vi "4_1_2.vi"() -> ()   [LabVIEW 2025, in "2022.lvlib"]
uses:
  2022.lvlib
  e0d1e511-853d-49ec-a1d4-7fdb9e36fbb4.vi
panel:
  out "size(s) 2":i32
  out "Array 4":bool[](array[boolean])
  out "size(s)":i32
  out "Array 3":bool[](array[boolean])
  out "x .or. y?":bool
  out "intersection":set{i32}(c389)
  out "Array 2":i32[](array[numeric])
  out "Array":i32[](array[numeric])
  out "output 4":i32
  out "output 3":i32
  out "output 2":i32
  out "output 1":i32
  out "subarray":string[](array[string])
  out "array":string[][](array[string])
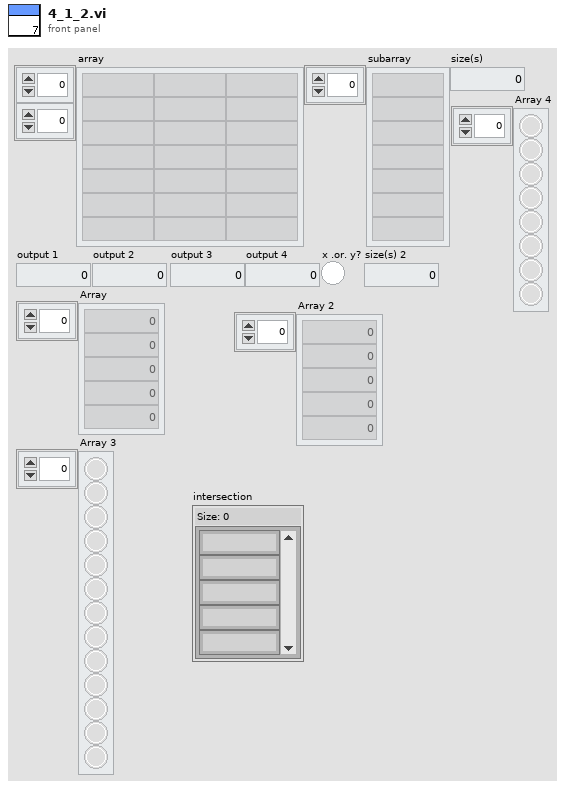
[diagram p1: front panel]
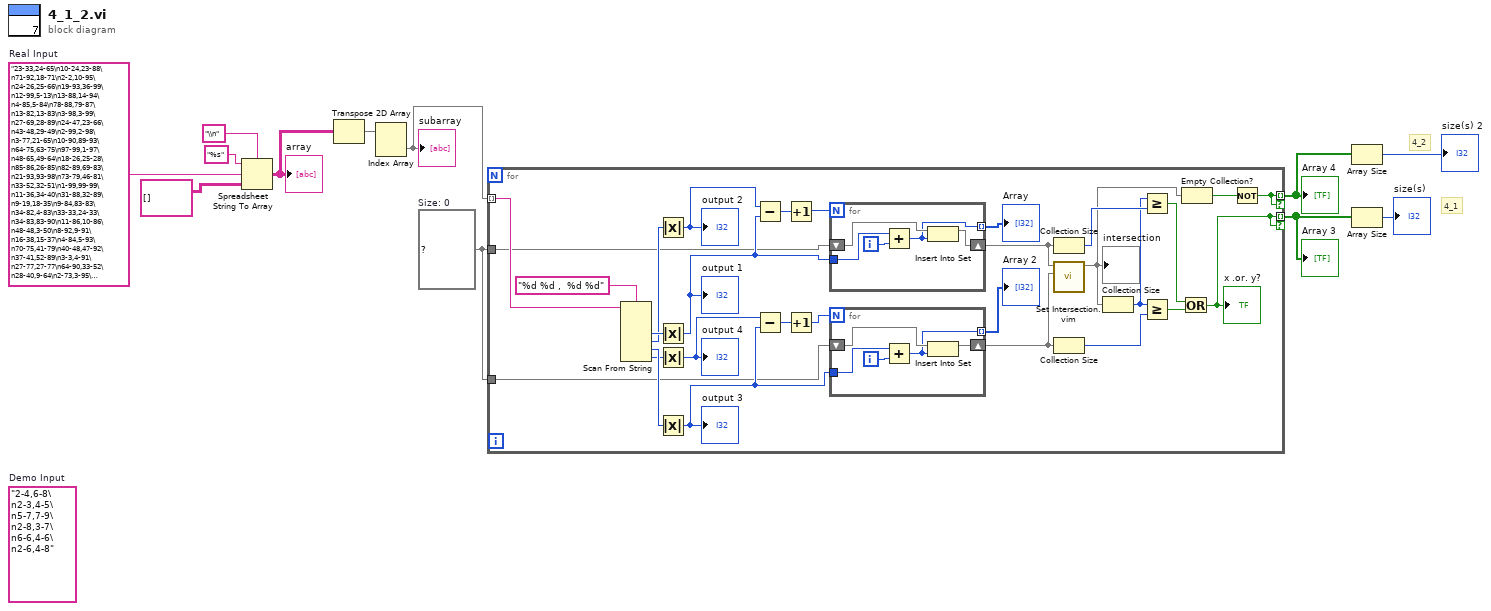
[diagram p0: block diagram]
diagram:
  w6 = set{i32} {}  # Size: 0
  w1 = "23-33,24-65\n10-24,23-88\n71-92,18-71\n2-2,10-95\n24-26,25-66\n19-93,36-99\n12-99,5-13\n13-88,14-94\n4-85,5-84\n78-88,79-87\n13-82,13-83\n3-98,3-99\n27-69,28-89\n24-47,23-66\n43-48,29-49\n2-99,2-98\n3-77,21-65\n10-90,89-93\n64-75,63-75\n97-99,1-97\n48-65,49-64\n18-26,25-28\n85-86,26-85\n82-89,69-83\n21-93,93-98\n73-79,46-81\n33-52,32-51\n1-99,99-99\n11-36,34-40\n31-88,32-89\n9-19,18-35\n9-84,83-83\n34-82,4-83\n33-33,24-33\n34-83,83-90\n11-86,10-86\n48-48,3-50\n8-92,9-91\n16-38,15-37\n4-84,5-93\n70-75,41-79\n40-48,47-92\n37-41,52-89\n3-3,4-91\n27-77,27-77\n64-90,33-52\n28-40,9-64\n2-73,3-95\n17-94,7-75\n6-71,7-71\n11-69,10-70\n4-40,4-40\n9-54,30-44\n92-93,4-92\n62-63,63-67\n7-34,16-34\n54-55,31-54\n12-90,11-91\n11-13,12-53\n10-73,9-64\n13-18,13-84\n6-82,16-81\n52-78,18-53\n22-82,23-74\n90-91,3-90\n92-93,70-93\n18-44,19-45\n20-20,20-67\n31-93,76-93\n25-86,86-86\n6-73,5-94\n75-84,74-86\n50-51,50-51\n56-86,57-86\n18-81,13-18\n3-9,8-93\n31-36,34-34\n19-88,18-87\n10-95,54-79\n83-85,66-86\n32-68,31-49\n14-97,12-99\n42-42,42-53\n27-32,28-69\n96-98,15-96\n25-49,25-48\n71-81,15-92\n19-83,15-19\n14-99,6-14\n52-90,53-94\n5-98,85-96\n18-30,10-15\n4-86,4-98\n54-55,30-78\n85-99,62-86\n10-99,10-98\n4-96,5-95\n6-59,7-18\n6-86,1-7\n28-85,5-84\n3-82,2-82\n73-92,87-87\n2-3,2-89\n4-5,4-8\n21-96,69-97\n89-90,4-89\n28-79,29-80\n35-58,40-48\n96-96,3-97\n17-27,16-96\n7-99,8-94\n26-92,25-92\n17-24,17-25\n44-44,40-47\n57-64,57-65\n60-91,59-79\n23-79,22-71\n34-37,31-70\n22-60,22-59\n44-99,98-98\n9-57,49-55\n61-64,33-62\n15-68,4-15\n53-55,34-55\n13-13,9-15\n2-43,3-81\n17-56,16-99\n1-4,3-92\n76-77,73-83\n2-97,2-96\n44-45,44-55\n8-89,8-97\n23-73,22-88\n23-90,79-93\n23-87,86-91\n3-45,17-44\n7-99,8-98\n92-97,14-92\n85-89,59-90\n7-8,7-89\n5-90,49-89\n28-30,29-63\n38-61,38-60\n32-98,5-75\n22-87,71-76\n5-85,5-88\n16-96,18-88\n39-51,40-90\n21-21,19-23\n22-55,15-56\n1-75,35-59\n13-84,12-85\n11-83,23-27\n11-98,11-97\n35-92,34-92\n8-96,8-30\n48-72,33-60\n9-83,10-82\n97-97,10-98\n5-7,9-98\n1-44,3-43\n7-85,8-85\n12-32,12-52\n1-86,86-86\n3-63,4-63\n3-83,83-91\n74-88,38-74\n92-95,6-98\n11-19,10-20\n6-94,7-94\n39-90,38-42\n60-92,61-92\n43-94,44-98\n23-98,22-99\n31-41,27-32\n9-79,9-78\n63-64,11-64\n82-82,83-98\n78-79,77-78\n19-63,4-27\n26-62,27-44\n91-91,91-93\n16-94,31-93\n23-25,24-99\n78-79,11-78\n30-30,29-31\n34-85,35-84\n4-78,4-5\n42-84,43-85\n39-87,40-86\n49-84,50-84\n67-67,7-67\n38-38,62-67\n2-83,3-82\n14-33,32-68\n18-76,17-75\n68-77,68-76\n4-97,53-73\n53-97,54-96\n53-55,54-98\n35-95,75-83\n2-3,2-78\n3-97,15-96\n26-87,26-92\n4-10,9-48\n3-89,22-96\n10-85,10-84\n1-93,2-2\n24-37,37-62\n32-68,48-53\n33-96,95-97\n9-26,14-31\n16-66,13-14\n85-86,78-85\n65-82,64-81\n5-85,31-49\n47-88,59-91\n34-71,70-76\n14-14,14-14\n45-46,45-97\n63-73,63-64\n16-54,17-53\n87-88,51-87\n20-79,19-98\n3-96,2-95\n86-86,60-86\n82-82,67-82\n12-35,11-35\n15-31,26-52\n1-2,1-99\n3-96,2-2\n91-97,11-92\n41-89,42-96\n62-64,41-65\n54-54,16-55\n28-41,40-97\n15-89,89-90\n50-71,55-70\n30-66,30-93\n89-92,84-89\n25-27,26-84\n59-91,60-91\n4-11,4-98\n5-48,10-44\n53-80,77-79\n20-21,10-20\n14-86,14-85\n32-70,33-69\n94-94,26-95\n5-57,5-97\n38-50,38-92\n48-50,49-51\n13-98,12-98\n90-95,24-88\n90-94,67-91\n1-11,10-91\n48-59,59-91\n26-68,31-55\n15-56,21-57\n6-69,7-69\n6-8,5-95\n32-93,33-94\n13-73,14-42\n1-4,3-98\n30-62,29-62\n57-64,61-99\n12-27,11-46\n28-99,98-98\n7-83,8-92\n56-77,56-76\n30-89,31-51\n69-83,37-72\n11-78,11-65\n61-61,60-62\n38-65,65-66\n20-44,21-97\n39-76,40-75\n10-94,11-93\n33-90,89-96\n23-77,22-78\n63-86,62-73\n42-81,35-43\n34-91,34-55\n12-97,4-13\n1-98,1-97\n23-72,24-73\n14-99,13-99\n17-97,18-96\n65-85,14-66\n68-77,67-69\n8-96,9-9\n28-57,29-56\n14-26,14-26\n6-72,6-72\n49-49,1-48\n4-65,65-65\n53-92,54-91\n48-87,15-48\n51-54,20-72\n65-75,64-64\n4-92,3-93\n42-70,30-98\n15-71,14-15\n29-62,28-63\n6-92,6-93\n37-84,83-83\n1-99,23-98\n23-82,24-88\n2-60,61-74\n3-5,17-93\n50-63,51-62\n51-55,52-52\n30-82,5-83\n5-77,4-42\n44-99,3-99\n18-81,5-18\n2-32,32-32\n50-59,58-87\n23-30,24-40\n70-70,9-71\n40-62,49-62\n2-29,1-3\n48-69,48-49\n48-48,47-93\n5-42,17-41\n11-95,12-92\n9-66,8-65\n32-84,33-84\n16-69,15-99\n12-96,9-12\n69-91,68-70\n14-69,15-81\n96-99,50-96\n35-62,35-61\n6-22,22-60\n20-76,73-74\n4-21,4-22\n22-30,21-76\n5-90,1-6\n82-96,82-95\n18-31,19-71\n29-56,50-59\n11-21,1-61\n15-76,30-81\n1-1,2-83\n11-90,90-91\n40-90,40-41\n68-83,68-83\n25-81,25-81\n87-88,22-87\n31-65,32-64\n17-90,16-90\n11-65,11-12\n35-60,36-93\n5-93,4-94\n28-29,27-75\n12-38,37-45\n39-46,32-44\n12-89,12-97\n4-54,52-52\n5-94,94-94\n30-31,29-31\n18-82,74-76\n80-80,59-81\n3-65,54-54\n20-31,19-23\n82-87,32-82\n41-41,41-42\n6-6,6-81\n2-98,98-98\n84-94,6-95\n29-89,28-92\n27-30,28-34\n5-86,4-86\n32-96,50-96\n28-93,69-90\n75-75,27-82\n9-30,30-36\n76-76,61-77\n74-80,11-74\n48-61,48-60\n64-98,64-99\n83-87,5-88\n23-25,25-98\n55-55,39-55\n5-36,5-36\n45-57,46-85\n4-86,3-85\n19-58,20-58\n25-83,14-26\n27-74,27-27\n17-18,17-45\n81-88,62-84\n84-96,21-85\n3-81,1-2\n54-93,1-94\n1-1,3-66\n69-78,49-78\n47-93,47-93\n13-13,13-66\n18-78,18-73\n11-20,15-18\n52-99,51-99\n2-57,1-58\n9-97,10-97\n80-80,24-80\n33-77,34-47\n68-75,67-73\n20-95,19-95\n4-99,5-98\n8-85,7-85\n42-80,66-82\n22-47,31-47\n22-26,24-24\n4-98,38-44\n92-94,92-95\n82-92,71-94\n6-10,1-5\n3-92,1-92\n72-76,71-74\n6-69,7-69\n25-75,26-66\n15-51,15-63\n14-99,14-98\n7-89,6-70\n58-66,62-85\n7-11,15-23\n42-62,42-63\n1-4,4-91\n1-3,3-97\n49-79,48-80\n15-95,16-77\n6-99,5-99\n6-79,8-27\n47-69,46-68\n20-21,24-96\n13-71,60-92\n69-94,36-69\n66-86,33-67\n34-47,34-47\n4-4,4-93\n22-68,68-68\n42-90,43-90\n74-74,74-94\n3-72,3-62\n63-75,64-67\n16-48,7-48\n2-89,3-99\n2-98,3-97\n41-94,42-95\n45-93,44-98\n16-18,17-64\n69-70,47-69\n2-93,93-94\n65-94,66-95\n54-56,55-57\n5-92,2-92\n48-92,28-45\n67-68,48-67\n7-12,6-8\n7-8,6-8\n94-99,16-95\n13-49,14-48\n25-48,48-48\n6-51,7-18\n46-83,15-97\n34-57,34-58\n16-89,9-17\n41-74,41-42\n13-32,13-97\n90-99,99-99\n7-99,7-98\n78-79,63-78\n4-98,64-79\n49-75,50-80\n40-75,40-52\n14-72,6-14\n5-91,91-91\n27-55,27-27\n20-22,27-37\n35-71,34-96\n2-52,1-1\n3-87,2-87\n2-70,36-69\n38-90,39-89\n67-79,67-80\n5-77,77-78\n26-32,2-34\n10-43,43-85\n55-84,84-85\n24-59,24-58\n43-49,44-48\n60-81,59-80\n52-91,91-92\n44-62,42-63\n3-96,3-97\n29-45,30-45\n64-92,6-93\n89-96,4-90\n71-91,71-90\n50-64,60-63\n49-88,49-89\n18-98,18-90\n30-74,72-77\n32-88,4-76\n22-58,22-23\n5-71,5-18\n8-90,7-98\n4-78,4-79\n54-87,54-55\n3-91,3-92\n14-92,89-91\n41-95,42-42\n74-75,53-77\n12-90,3-12\n5-50,3-51\n27-67,66-68\n10-42,24-38\n20-79,20-81\n10-78,78-97\n26-47,35-46\n34-82,34-63\n2-94,3-98\n19-87,19-87\n4-42,6-90\n13-49,12-14\n75-75,3-76\n55-70,54-56\n86-92,85-93\n31-38,28-46\n7-90,6-91\n33-72,32-50\n22-46,45-99\n45-53,46-51\n90-91,6-90\n13-87,14-45\n41-95,14-42\n90-95,76-95\n51-70,15-89\n15-49,25-95\n15-15,15-98\n20-88,14-33\n2-67,67-70\n88-93,78-96\n77-91,53-84\n53-88,52-98\n24-96,25-25\n40-40,26-40\n3-15,9-25\n35-99,36-97\n61-61,4-62\n5-95,6-6\n52-56,52-95\n22-30,23-23\n40-44,43-63\n13-16,5-14\n18-90,89-89\n5-88,4-88\n78-83,82-82\n6-80,1-1\n15-31,14-32\n13-96,13-13\n68-76,68-69\n56-67,67-90\n24-92,92-93\n16-29,17-90\n2-99,1-90\n12-75,1-13\n21-91,20-90\n1-99,11-97\n94-94,25-95\n2-91,3-92\n95-95,2-95\n2-99,1-97\n28-98,27-29\n6-26,2-67\n20-58,19-71\n32-87,49-86\n13-57,14-56\n2-55,11-44\n13-61,12-61\n33-81,80-80\n39-91,41-44\n40-93,39-47\n83-95,40-93\n20-79,24-78\n52-93,6-94\n96-96,3-97\n44-55,36-87\n43-44,13-43\n19-99,19-98\n6-17,17-97\n91-99,88-91\n31-51,52-77\n1-97,1-2\n26-86,26-87\n50-53,40-81\n40-89,89-93\n78-83,1-79\n9-89,8-73\n6-38,7-21\n19-20,18-21\n97-97,35-97\n28-57,20-28\n3-86,86-87\n53-53,2-52\n59-99,60-99\n75-84,76-95\n20-93,21-94\n29-29,29-30\n34-92,15-58\n11-58,11-59\n11-11,10-98\n19-77,77-77\n38-56,38-71\n83-86,12-88\n8-73,5-6\n5-7,7-93\n18-79,19-72\n4-99,2-2\n5-82,5-81\n24-37,37-95\n11-63,9-12\n6-99,7-98\n92-92,91-91\n58-91,2-95\n23-98,24-59\n2-90,3-89\n54-71,1-81\n22-98,48-97\n14-49,13-76\n5-52,6-89\n6-88,76-86\n3-85,6-97\n87-94,86-88\n30-46,31-45\n63-95,9-97\n19-94,94-98\n71-75,72-74\n48-89,49-89\n27-52,52-54\n21-99,41-94\n5-96,3-5\n40-69,38-40\n74-99,73-98\n6-31,22-85\n13-76,12-75\n29-74,29-74\n10-86,11-86\n40-41,33-40\n63-94,29-94\n55-85,55-55\n14-20,18-19\n52-78,1-79\n92-96,7-92\n12-89,14-57\n32-49,49-82\n36-63,43-62\n20-94,41-93\n79-95,7-97\n5-60,5-22\n29-93,28-93\n18-68,18-67\n12-37,13-36\n12-64,12-46\n1-99,2-2\n61-92,61-82\n14-16,15-68\n68-83,67-77\n24-93,93-93\n33-99,32-33\n93-93,11-94\n27-37,26-37\n7-31,6-31\n1-45,2-67\n5-99,5-99\n20-21,18-22\n22-89,23-88\n53-58,53-56\n48-91,48-86\n11-11,10-12\n33-50,50-81\n11-47,7-20\n51-71,71-72\n15-89,15-88\n6-90,2-15\n7-88,18-91\n4-98,4-98\n9-19,3-19\n29-58,57-83\n16-34,15-33\n13-50,12-89\n17-60,17-17\n90-94,91-98\n52-77,52-76\n97-99,5-97\n42-86,53-76\n4-7,19-56\n23-63,2-41\n15-43,43-44\n19-23,22-97\n47-48,45-49\n31-73,32-73\n57-72,21-38\n54-97,53-96\n2-29,3-64\n53-79,13-77\n63-77,4-63\n94-94,4-95\n5-44,4-98\n5-99,4-98\n31-96,32-96\n44-89,43-90\n1-63,2-63\n31-60,8-32\n48-88,55-62\n36-85,35-85\n7-98,97-97\n3-52,4-99\n19-57,1-20\n65-96,66-97\n61-95,43-62\n4-94,93-93\n14-97,58-96\n26-46,6-47\n79-96,81-95\n30-88,30-87\n27-97,26-96\n24-88,24-25\n27-95,28-51\n22-24,23-76\n40-44,44-52\n4-37,3-38\n6-7,4-8\n22-24,16-25\n59-73,58-73\n2-14,3-40\n20-65,65-65\n58-87,58-86\n99-99,26-98\n10-17,16-91\n52-71,59-70\n3-87,2-87\n22-95,95-96\n55-55,10-54\n52-84,82-96\n5-82,81-81\n9-95,7-7\n53-88,88-90\n5-6,5-63\n11-68,10-85\n8-12,10-11\n40-92,43-49\n19-35,20-34\n44-46,45-85\n10-25,12-26\n63-85,54-80\n10-97,91-94\n41-50,40-42\n7-72,8-71\n1-15,12-92\n22-93,54-99\n82-94,30-83\n7-89,6-89\n6-69,5-7\n8-25,24-24\n8-47,8-47\n21-25,24-92\n81-81,81-86\n6-15,44-68\n82-82,34-82\n29-86,2-87\n37-54,20-57\n56-97,1-96\n65-65,6-65\n4-81,5-82\n78-85,37-78\n18-99,19-97\n31-97,34-96\n41-58,40-77\n11-96,10-97\n18-35,7-24\n5-75,3-74\n2-53,15-47\n9-17,9-85\n20-26,21-26\n23-70,67-68\n23-72,23-73\n36-81,9-93\n25-76,25-26\n77-77,46-77\n78-98,78-87\n91-91,14-92\n22-92,21-93\n3-3,3-87\n99-99,61-99\n18-28,19-29\n44-45,19-44\n17-60,11-17\n35-97,36-36\n58-58,11-58\n24-62,23-63\n18-56,55-81\n7-31,8-30\n60-61,1-65\n8-99,7-31\n2-4,5-6\n4-93,48-92\n2-87,1-98\n3-75,3-4\n1-53,53-54\n57-73,57-68\n11-60,2-61\n51-70,43-52\n4-33,3-34\n29-68,67-68\n75-86,28-71\n4-84,3-83\n12-96,51-96\n30-98,71-94\n54-62,60-62\n13-66,14-86\n14-42,12-43\n47-69,48-69\n58-89,86-96\n27-96,27-95\n6-66,6-16\n2-30,1-37\n27-91,27-38\n46-52,45-49\n9-64,8-75\n53-92,54-93\n35-91,35-72\n66-91,91-97\n46-81,49-81\n3-90,1-3\n53-54,52-56\n4-92,3-5\n42-84,42-77\n1-3,2-95\n8-73,9-90\n17-69,16-70\n9-20,2-10\n97-99,96-97\n1-86,2-91\n17-66,9-95\n9-10,9-97\n19-40,39-54\n5-94,5-91\n33-33,18-34\n2-3,2-3\n22-66,21-84\n37-90,37-81\n6-93,6-93\n64-81,65-78\n57-59,57-67\n69-94,68-68\n39-97,38-98\n74-79,71-79\n2-80,41-80\n5-91,28-89\n1-97,2-97\n24-61,25-94\n76-81,76-97\n48-56,48-49\n25-81,7-12\n42-99,41-41\n45-60,46-59\n19-85,57-84\n8-8,7-98\n14-53,13-54\n17-82,69-84\n73-86,24-90\n78-80,6-78\n2-76,3-26\n1-33,33-89\n12-48,48-75\n25-87,21-88\n22-68,22-71\n2-91,1-91\n59-79,7-60\n6-70,4-4\n47-94,27-94\n23-50,10-49\n2-85,2-83\n2-96,7-96\n21-93,22-92\n27-67,28-67\n32-38,32-33\n15-94,93-94\n36-74,36-37\n33-84,43-83\n5-98,2-2\n1-93,2-92\n37-97,42-70\n81-82,21-81\n14-94,13-15\n5-45,4-87\n44-96,45-95\n2-7,6-14\n14-73,25-77\n83-83,84-99\n13-62,21-73\n91-98,22-91\n19-96,86-93\n5-78,6-77\n3-97,4-98\n8-54,17-83\n9-94,10-10\n36-96,35-37\n8-93,7-98\n48-60,48-61\n17-97,9-18\n73-87,74-88\n19-63,19-63\n21-73,20-74\n1-89,26-89\n44-50,48-55\n43-70,70-71\n5-14,6-63\n23-82,22-94\n20-67,18-94\n36-52,47-51\n10-84,9-83\n18-96,18-71\n3-64,4-65\n4-7,6-89\n62-89,73-99\n4-92,3-5\n3-62,45-59\n9-98,10-97\n12-80,12-89\n14-15,18-85\n7-18,6-23\n14-70,15-24\n24-52,21-78\n63-92,32-93\n47-91,42-48\n16-91,91-95\n31-66,30-65\n52-91,5-91\n85-85,11-86\n22-69,68-68\n11-58,10-21\n47-76,42-47\n63-64,43-66\n17-29,4-66\n19-19,18-86\n33-70,33-70\n33-38,32-38\n3-5,4-99\n14-55,13-55\n4-48,4-4\n80-96,79-98\n99-99,5-29\n48-72,49-72\n5-91,3-92\n10-25,10-26\n9-11,10-28\n29-39,28-38\n19-55,55-56\n1-14,1-2\n21-81,21-81\n32-89,38-86\n31-79,31-39\n66-72,67-73\n3-3,2-29\n9-67,10-10\n24-96,23-25\n90-94,90-93\n91-91,7-92\n45-98,44-93\n1-76,3-75\n14-59,22-60\n12-70,4-21\n30-93,25-98\n18-30,9-19\n1-4,3-90\n9-95,9-22\n92-96,59-92\n26-67,22-25\n7-9,8-30\n74-82,82-83\n92-92,4-93\n14-76,2-63\n52-86,51-82\n11-98,10-12\n2-97,96-96\n18-91,18-99\n15-36,17-92\n14-90,13-91\n14-88,87-99\n47-92,48-92\n3-97,10-93\n9-87,80-98\n4-96,3-5\n89-99,3-89\n11-65,10-66\n4-52,52-93\n29-31,12-28"  # Real Input
  (unwired) "2-4,6-8\n2-3,4-5\n5-7,7-9\n2-8,3-7\n6-6,4-6\n2-6,4-8"  # Demo Input
  # "4_2"
  # "4_1"
  n1 = Spreadsheet String To Array(delimiter (Tab)="\\n", format string="%s" ("delimiter"), spreadsheet string=w1, array type (2D Dbl)=string[][] []) -> (array=w9:string[][])
  "array" <- w9
  n2 = Transpose 2D Array(2D array=w9) -> (transposed array=w8:string[][])
  n3 = Index Array(array=w8) -> (element=w7:string[])  [unwired: 2 in]
  "subarray" <- w7
  n4 = for {
    tunnel: w7 -> [w41] mode=indexing
    tunnel: w6 -> [w27]
    tunnel: w6 -> [w26]
    tunnel: [w16] -> w5 mode=indexing if=w16
    tunnel: [w13] -> w3 mode=indexing if=w13
    n5 = Scan From String(format string="%d %d ,  %d %d", input string=w41) -> (output 1=w39:i32, output 2=w38:i32, output 3=w37:i32, output 4=w36:i32)  [unwired: 6 in, 3 out]
    n6 = Absolute Value(x=w38) -> (abs(x)=w25:i32)
    "output 2" <- w25
    n7 = Absolute Value(x=w39) -> (abs(x)=w33:i32)
    "output 1" <- w33
    n8 = Absolute Value(x=w36) -> (abs(x)=w24:i32)
    "output 4" <- w24
    n9 = Absolute Value(x=w37) -> (abs(x)=w29:i32)
    "output 3" <- w29
    n10 = Subtract(x=w25, y=w33) -> (x-y=w35:i32)
    n11 = Subtract(x=w24, y=w29) -> (x-y=w31:i32)
    n12 = Increment(x=w35) -> (x+1=w34:i32)
    n13 = Increment(x=w31) -> (x+1=w30:i32)
    n14 = for {
      N: w34 -> [_]
      tunnel: w33 -> [w50]
      tunnel: [w48] -> w32 mode=indexing
      shift-right: [w47] -> w22
      shift-left: w27 -> [w49]
      i -> [w51]
      n15 = Add(x=w50, y=w51) -> (x+y=w48:i32)
      n16 = Insert Into Set(10:w48, 11:w49) -> (3:w47:set{i32})  [unwired: 1 out]
    }
    "Array" <- w32
    n17 = for {
      N: w30 -> [_]
      tunnel: w29 -> [w45]
      tunnel: [w42] -> w28 mode=indexing
      shift-right: [w43] -> w23
      shift-left: w26 -> [w44]
      i -> [w46]
      n18 = Add(x=w45, y=w46) -> (x+y=w42:i32)
      n19 = Insert Into Set(10:w42, 11:w44) -> (3:w43:set{i32})  [unwired: 1 out]
    }
    "Array 2" <- w28
    n20 = Collection Size(1:w22) -> (0:w21:i32)
    n21 = call "Set Intersection.vim"("set 2"=w23, "set 1"=w22) -> ("intersection"=w15:set{i32})  [unwired: 9 in]
    "intersection" <- w15
    n22 = Collection Size(1:w23) -> (0:w18:i32)
    n23 = Collection Size(1:w15) -> (0:w19:i32)
    n24 = Greater Or Equal?(x=w19, y=w21) -> (x >= y?=w20:bool)
    n25 = Greater Or Equal?(x=w19, y=w18) -> (x >= y?=w17:bool)
    n26 = Or(x=w20, y=w17) -> (x .or. y?=w16:bool)
    "x .or. y?" <- w16
    n27 = Empty Collection?(1:w15) -> (0:w14:bool)
    n28 = Not(x=w14) -> (.not. x?=w13:bool)
  }
  "Array 3" <- w5
  "Array 4" <- w3
  n29 = Array Size(array=w3) -> (size(s)=→"size(s) 2":i32)
  n30 = Array Size(array=w5) -> (size(s)=→"size(s)":i32)
